vi "set lights for given state.vi"(7 "light state":T1) -> (8 "all lights out":T2)   [LabVIEW 2016]
doc: "This vi sets the particular light on/off configuration for all of the lights in the intersection state machine appropriate to a particular state.\n\nAlexis Lopez\nP350\nCSUSB Physics"
uses:
  typedefs/all lights.ctl
  typedefs/light set.ctl
  typedefs/stop light.ctl
  typedefs/left arrow.ctl
  typedefs/walk light.ctl
  typedefs/state enum.ctl
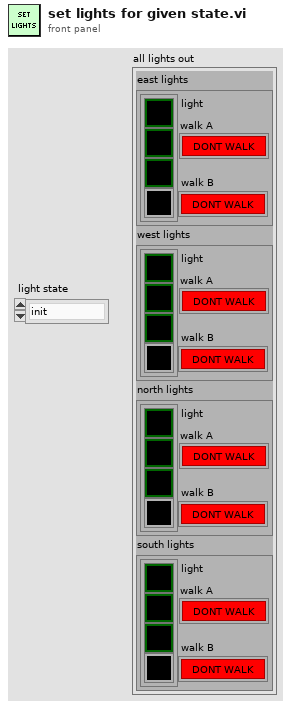
[diagram p1: front panel]
types:
  T1 = typedef "state enum.ctl" = enum16{"init", "idle", "left turn E", "go EW", "caution EW", "left turn W", "left turn N", "go NS", "caution NS", "left turn S", "blink on", "blink off", "all on test", "exit"}
  T2 = typedef "all lights.ctl" = cluster{"east lights":T3, "west lights":T3, "north lights":T3, "south lights":T3}
  T3 = typedef "light set.ctl" = cluster{"light":T4, "walk A":T6, "walk B":T6}
  T4 = typedef "stop light.ctl" = cluster{"stop":bool, "caution":bool, "go":bool, "arrow":T5}
  T5 = typedef "left arrow.ctl" = bool
  T6 = typedef "walk light.ctl" = bool
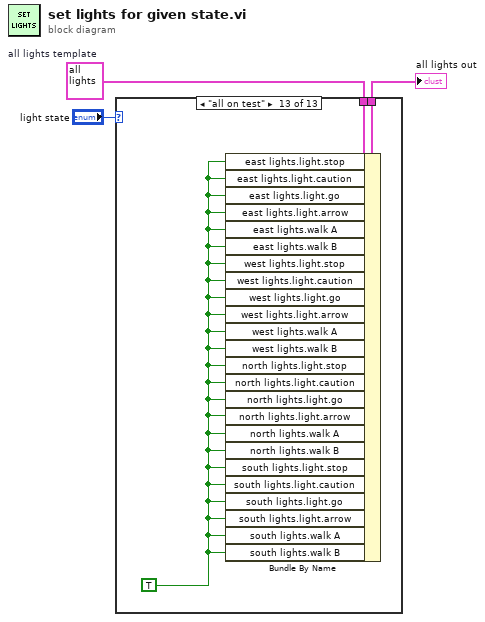
[diagram p0: block diagram]
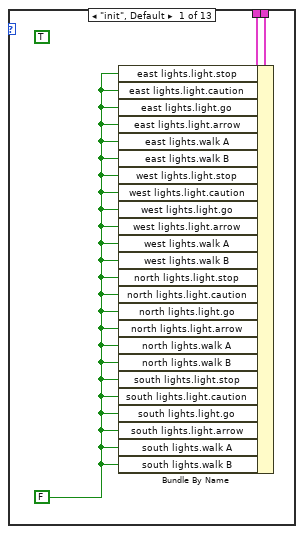
[diagram p2: hidden frame]
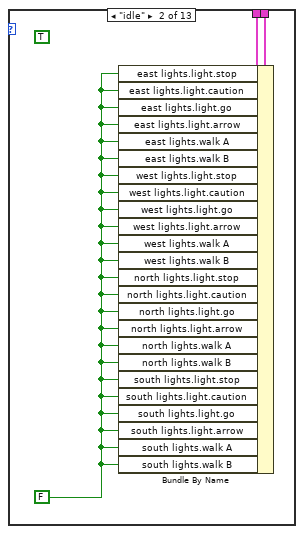
[diagram p3: hidden frame]
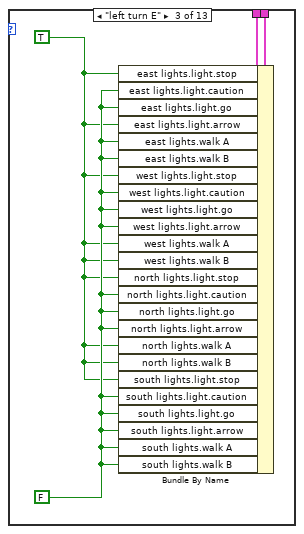
[diagram p4: hidden frame]
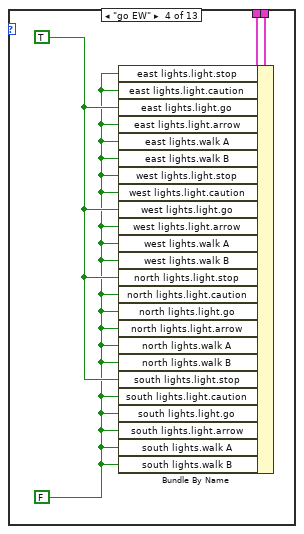
[diagram p5: hidden frame]
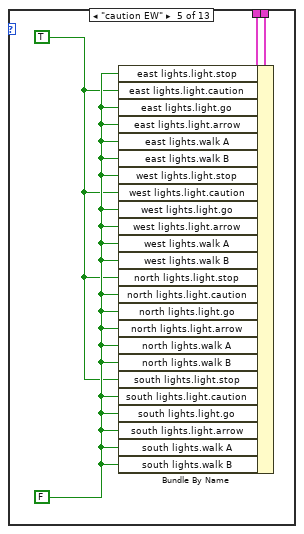
[diagram p6: hidden frame]
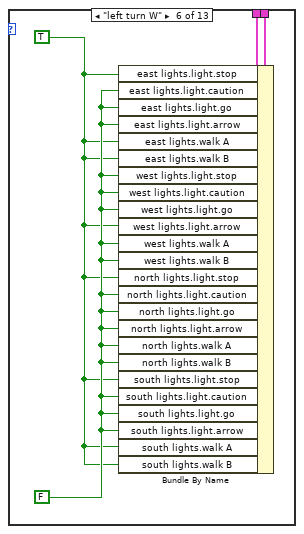
[diagram p7: hidden frame]
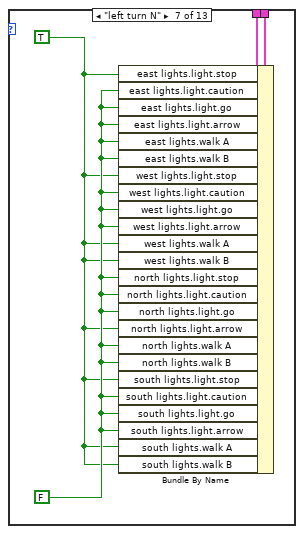
[diagram p8: hidden frame]
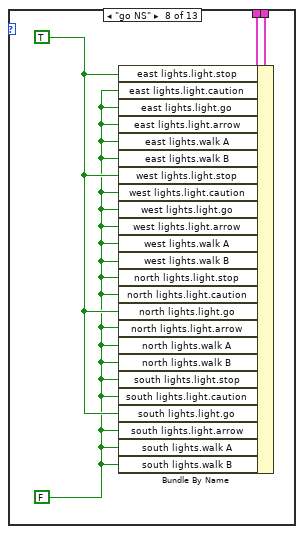
[diagram p9: hidden frame]
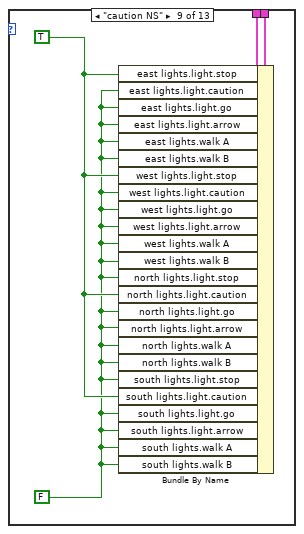
[diagram p10: hidden frame]
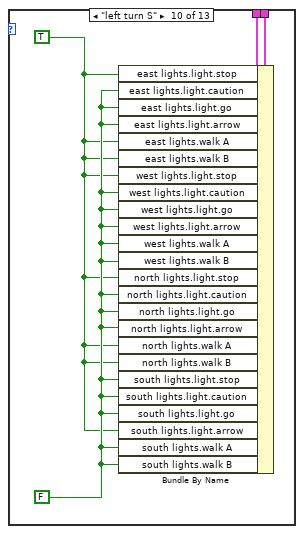
[diagram p11: hidden frame]
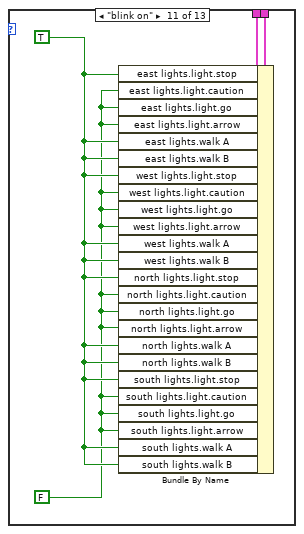
[diagram p12: hidden frame]
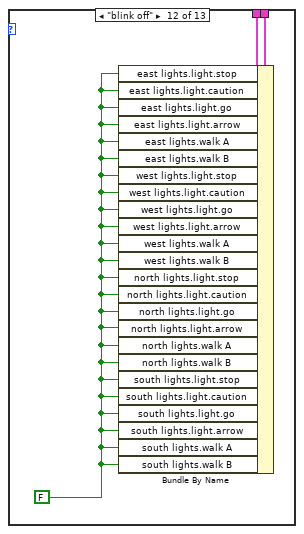
[diagram p13: hidden frame]
diagram:
  w2 = T2 {"east lights"={"light"={"stop"=FALSE, "caution"=FALSE, "go"=FALSE, "arrow"=FALSE}, "walk A"=FALSE, "walk B"=FALSE}, "west lights"={"light"={"stop"=FALSE, "caution"=FALSE, "go"=FALSE, "arrow"=FALSE}, "walk A"=FALSE, "walk B"=FALSE}, "north lights"={"light"={"stop"=FALSE, "caution"=FALSE, "go"=FALSE, "arrow"=FALSE}, "walk A"=FALSE, "walk B"=FALSE}, "south lights"={"light"={"stop"=FALSE, "caution"=FALSE, "go"=FALSE, "arrow"=FALSE}, "walk A"=FALSE, "walk B"=FALSE}}  # all lights template
  n1 = case shown="\"all on test\"" "light state" {
    tunnel: w2 -> [w6 w9 w13 w17 w21 w25 w29 w33 w37 w41 w45 w48 w51]
    tunnel: [w5 w8 w12 w16 w20 w24 w28 w32 w36 w40 w44 w47 w50] -> w1
    frame "init", Default {
      (unwired) TRUE
      w4 = FALSE
      n2 = Bundle By Name(cluster=w6, "east lights.light.stop"=w4, "east lights.light.caution"=w4, "east lights.light.go"=w4, "east lights.light.arrow"=w4, "east lights.walk A"=w4, "east lights.walk B"=w4, "west lights.light.stop"=w4, "west lights.light.caution"=w4, "west lights.light.go"=w4, "west lights.light.arrow"=w4, "west lights.walk A"=w4, "west lights.walk B"=w4, "north lights.light.stop"=w4, "north lights.light.caution"=w4, "north lights.light.go"=w4, "north lights.light.arrow"=w4, "north lights.walk A"=w4, "north lights.walk B"=w4, "south lights.light.stop"=w4, "south lights.light.caution"=w4, "south lights.light.go"=w4, "south lights.light.arrow"=w4, "south lights.walk A"=w4, "south lights.walk B"=w4) -> (w5:T2)
    }
    frame "idle" {
      (unwired) TRUE
      w7 = FALSE
      n3 = Bundle By Name(cluster=w9, "east lights.light.stop"=w7, "east lights.light.caution"=w7, "east lights.light.go"=w7, "east lights.light.arrow"=w7, "east lights.walk A"=w7, "east lights.walk B"=w7, "west lights.light.stop"=w7, "west lights.light.caution"=w7, "west lights.light.go"=w7, "west lights.light.arrow"=w7, "west lights.walk A"=w7, "west lights.walk B"=w7, "north lights.light.stop"=w7, "north lights.light.caution"=w7, "north lights.light.go"=w7, "north lights.light.arrow"=w7, "north lights.walk A"=w7, "north lights.walk B"=w7, "south lights.light.stop"=w7, "south lights.light.caution"=w7, "south lights.light.go"=w7, "south lights.light.arrow"=w7, "south lights.walk A"=w7, "south lights.walk B"=w7) -> (w8:T2)
    }
    frame "left turn E" {
      w10 = TRUE
      w11 = FALSE
      n4 = Bundle By Name(cluster=w13, "east lights.light.stop"=w10, "east lights.light.caution"=w11, "east lights.light.go"=w11, "east lights.light.arrow"=w10, "east lights.walk A"=w11, "east lights.walk B"=w11, "west lights.light.stop"=w10, "west lights.light.caution"=w11, "west lights.light.go"=w11, "west lights.light.arrow"=w11, "west lights.walk A"=w10, "west lights.walk B"=w10, "north lights.light.stop"=w10, "north lights.light.caution"=w11, "north lights.light.go"=w11, "north lights.light.arrow"=w11, "north lights.walk A"=w10, "north lights.walk B"=w10, "south lights.light.stop"=w10, "south lights.light.caution"=w11, "south lights.light.go"=w11, "south lights.light.arrow"=w11, "south lights.walk A"=w11, "south lights.walk B"=w11) -> (w12:T2)
    }
    frame "go EW" {
      w15 = TRUE
      w14 = FALSE
      n5 = Bundle By Name(cluster=w17, "east lights.light.stop"=w14, "east lights.light.caution"=w14, "east lights.light.go"=w15, "east lights.light.arrow"=w14, "east lights.walk A"=w14, "east lights.walk B"=w14, "west lights.light.stop"=w14, "west lights.light.caution"=w14, "west lights.light.go"=w15, "west lights.light.arrow"=w14, "west lights.walk A"=w14, "west lights.walk B"=w14, "north lights.light.stop"=w15, "north lights.light.caution"=w14, "north lights.light.go"=w14, "north lights.light.arrow"=w14, "north lights.walk A"=w14, "north lights.walk B"=w14, "south lights.light.stop"=w15, "south lights.light.caution"=w14, "south lights.light.go"=w14, "south lights.light.arrow"=w14, "south lights.walk A"=w14, "south lights.walk B"=w14) -> (w16:T2)
    }
    frame "caution EW" {
      w18 = TRUE
      w19 = FALSE
      n6 = Bundle By Name(cluster=w21, "east lights.light.stop"=w19, "east lights.light.caution"=w18, "east lights.light.go"=w19, "east lights.light.arrow"=w19, "east lights.walk A"=w19, "east lights.walk B"=w19, "west lights.light.stop"=w19, "west lights.light.caution"=w18, "west lights.light.go"=w19, "west lights.light.arrow"=w19, "west lights.walk A"=w19, "west lights.walk B"=w19, "north lights.light.stop"=w18, "north lights.light.caution"=w19, "north lights.light.go"=w19, "north lights.light.arrow"=w19, "north lights.walk A"=w19, "north lights.walk B"=w19, "south lights.light.stop"=w18, "south lights.light.caution"=w19, "south lights.light.go"=w19, "south lights.light.arrow"=w19, "south lights.walk A"=w19, "south lights.walk B"=w19) -> (w20:T2)
    }
    frame "left turn W" {
      w22 = TRUE
      w23 = FALSE
      n7 = Bundle By Name(cluster=w25, "east lights.light.stop"=w22, "east lights.light.caution"=w23, "east lights.light.go"=w23, "east lights.light.arrow"=w23, "east lights.walk A"=w22, "east lights.walk B"=w22, "west lights.light.stop"=w23, "west lights.light.caution"=w23, "west lights.light.go"=w23, "west lights.light.arrow"=w22, "west lights.walk A"=w23, "west lights.walk B"=w23, "north lights.light.stop"=w22, "north lights.light.caution"=w23, "north lights.light.go"=w23, "north lights.light.arrow"=w23, "north lights.walk A"=w23, "north lights.walk B"=w23, "south lights.light.stop"=w22, "south lights.light.caution"=w23, "south lights.light.go"=w23, "south lights.light.arrow"=w23, "south lights.walk A"=w22, "south lights.walk B"=w22) -> (w24:T2)
    }
    frame "left turn N" {
      w26 = TRUE
      w27 = FALSE
      n8 = Bundle By Name(cluster=w29, "east lights.light.stop"=w26, "east lights.light.caution"=w27, "east lights.light.go"=w27, "east lights.light.arrow"=w27, "east lights.walk A"=w27, "east lights.walk B"=w27, "west lights.light.stop"=w26, "west lights.light.caution"=w27, "west lights.light.go"=w27, "west lights.light.arrow"=w27, "west lights.walk A"=w26, "west lights.walk B"=w26, "north lights.light.stop"=w27, "north lights.light.caution"=w27, "north lights.light.go"=w27, "north lights.light.arrow"=w26, "north lights.walk A"=w27, "north lights.walk B"=w27, "south lights.light.stop"=w26, "south lights.light.caution"=w27, "south lights.light.go"=w27, "south lights.light.arrow"=w27, "south lights.walk A"=w26, "south lights.walk B"=w26) -> (w28:T2)
    }
    frame "go NS" {
      w31 = TRUE
      w30 = FALSE
      n9 = Bundle By Name(cluster=w33, "east lights.light.stop"=w31, "east lights.light.caution"=w30, "east lights.light.go"=w30, "east lights.light.arrow"=w30, "east lights.walk A"=w30, "east lights.walk B"=w30, "west lights.light.stop"=w31, "west lights.light.caution"=w30, "west lights.light.go"=w30, "west lights.light.arrow"=w30, "west lights.walk A"=w30, "west lights.walk B"=w30, "north lights.light.stop"=w30, "north lights.light.caution"=w30, "north lights.light.go"=w31, "north lights.light.arrow"=w30, "north lights.walk A"=w30, "north lights.walk B"=w30, "south lights.light.stop"=w30, "south lights.light.caution"=w30, "south lights.light.go"=w31, "south lights.light.arrow"=w30, "south lights.walk A"=w30, "south lights.walk B"=w30) -> (w32:T2)
    }
    frame "caution NS" {
      w35 = TRUE
      w34 = FALSE
      n10 = Bundle By Name(cluster=w37, "east lights.light.stop"=w35, "east lights.light.caution"=w34, "east lights.light.go"=w34, "east lights.light.arrow"=w34, "east lights.walk A"=w34, "east lights.walk B"=w34, "west lights.light.stop"=w35, "west lights.light.caution"=w34, "west lights.light.go"=w34, "west lights.light.arrow"=w34, "west lights.walk A"=w34, "west lights.walk B"=w34, "north lights.light.stop"=w34, "north lights.light.caution"=w35, "north lights.light.go"=w34, "north lights.light.arrow"=w34, "north lights.walk A"=w34, "north lights.walk B"=w34, "south lights.light.stop"=w34, "south lights.light.caution"=w35, "south lights.light.go"=w34, "south lights.light.arrow"=w34, "south lights.walk A"=w34, "south lights.walk B"=w34) -> (w36:T2)
    }
    frame "left turn S" {
      w38 = TRUE
      w39 = FALSE
      n11 = Bundle By Name(cluster=w41, "east lights.light.stop"=w38, "east lights.light.caution"=w39, "east lights.light.go"=w39, "east lights.light.arrow"=w39, "east lights.walk A"=w38, "east lights.walk B"=w38, "west lights.light.stop"=w38, "west lights.light.caution"=w39, "west lights.light.go"=w39, "west lights.light.arrow"=w39, "west lights.walk A"=w39, "west lights.walk B"=w39, "north lights.light.stop"=w38, "north lights.light.caution"=w39, "north lights.light.go"=w39, "north lights.light.arrow"=w39, "north lights.walk A"=w38, "north lights.walk B"=w38, "south lights.light.stop"=w39, "south lights.light.caution"=w39, "south lights.light.go"=w39, "south lights.light.arrow"=w38, "south lights.walk A"=w39, "south lights.walk B"=w39) -> (w40:T2)
    }
    frame "blink on" {
      w43 = TRUE
      w42 = FALSE
      n12 = Bundle By Name(cluster=w45, "east lights.light.stop"=w43, "east lights.light.caution"=w42, "east lights.light.go"=w42, "east lights.light.arrow"=w42, "east lights.walk A"=w43, "east lights.walk B"=w43, "west lights.light.stop"=w43, "west lights.light.caution"=w42, "west lights.light.go"=w42, "west lights.light.arrow"=w42, "west lights.walk A"=w43, "west lights.walk B"=w43, "north lights.light.stop"=w43, "north lights.light.caution"=w42, "north lights.light.go"=w42, "north lights.light.arrow"=w42, "north lights.walk A"=w43, "north lights.walk B"=w43, "south lights.light.stop"=w43, "south lights.light.caution"=w42, "south lights.light.go"=w42, "south lights.light.arrow"=w42, "south lights.walk A"=w43, "south lights.walk B"=w43) -> (w44:T2)
    }
    frame "blink off" {
      w46 = FALSE
      n13 = Bundle By Name(cluster=w48, "east lights.light.stop"=w46, "east lights.light.caution"=w46, "east lights.light.go"=w46, "east lights.light.arrow"=w46, "east lights.walk A"=w46, "east lights.walk B"=w46, "west lights.light.stop"=w46, "west lights.light.caution"=w46, "west lights.light.go"=w46, "west lights.light.arrow"=w46, "west lights.walk A"=w46, "west lights.walk B"=w46, "north lights.light.stop"=w46, "north lights.light.caution"=w46, "north lights.light.go"=w46, "north lights.light.arrow"=w46, "north lights.walk A"=w46, "north lights.walk B"=w46, "south lights.light.stop"=w46, "south lights.light.caution"=w46, "south lights.light.go"=w46, "south lights.light.arrow"=w46, "south lights.walk A"=w46, "south lights.walk B"=w46) -> (w47:T2)
    }
    frame "all on test" {
      w49 = TRUE
      n14 = Bundle By Name(cluster=w51, "east lights.light.stop"=w49, "east lights.light.caution"=w49, "east lights.light.go"=w49, "east lights.light.arrow"=w49, "east lights.walk A"=w49, "east lights.walk B"=w49, "west lights.light.stop"=w49, "west lights.light.caution"=w49, "west lights.light.go"=w49, "west lights.light.arrow"=w49, "west lights.walk A"=w49, "west lights.walk B"=w49, "north lights.light.stop"=w49, "north lights.light.caution"=w49, "north lights.light.go"=w49, "north lights.light.arrow"=w49, "north lights.walk A"=w49, "north lights.walk B"=w49, "south lights.light.stop"=w49, "south lights.light.caution"=w49, "south lights.light.go"=w49, "south lights.light.arrow"=w49, "south lights.walk A"=w49, "south lights.walk B"=w49) -> (w50:T2)
    }
  }
  "all lights out" <- w1
